vi "ageing subrutine test6.vi"() -> ()   [LabVIEW 2011]
uses:
  <vilib>/Utility/miscctls.llb/LVRowAndColumnTypeDef.ctl
  Controls Win/Control 3.ctl
  <vilib>/Utility/file.llb/Write To Spreadsheet File (string).vi
  <vilib>/Utility/file.llb/Read From Spreadsheet File (string).vi
  <vilib>/regexp/Match Regular Expression.xnode
panel:
  out "Flag 2":bool=TRUE
  out "Flag1":bool=TRUE
  out "Ageing array":string[](array[string])
  out "EditPos Subc":T1
  in  "Ageing Gas":enum32{"Radio Selection 1", "Radio Selection 2"}(radio)
  out "Total Test Duration (Hr)":string
  in  "Clear Pattern":bool
  in  "Clear Pattern":bool
  in  "Subcycle name":string
  in  "Subcycle Pattern":string[][](table) caption="Subcycle pattern"
  in  "stop":bool
  out "Cycle Compiled":bool
  in  "Load cycle for test":bool
  in  "Cycle name":string
  in  "Cycle List":i32(listbox)=2
  in  "Delete Cycle":bool
  in  "Load Cycle":bool
  in  "Save Cycle":bool
  in  "Delete Subcycle":bool
  in  "Subcycle List":i32(listbox)=1
  in  "Load Subcycle":bool
  in  "Save Subcycle":bool
  in  "Cycle Pattern":string[][](table)
  in  "Total Number of Cycles":dbl=1.0 min=1.0
  # "Ageing Program"
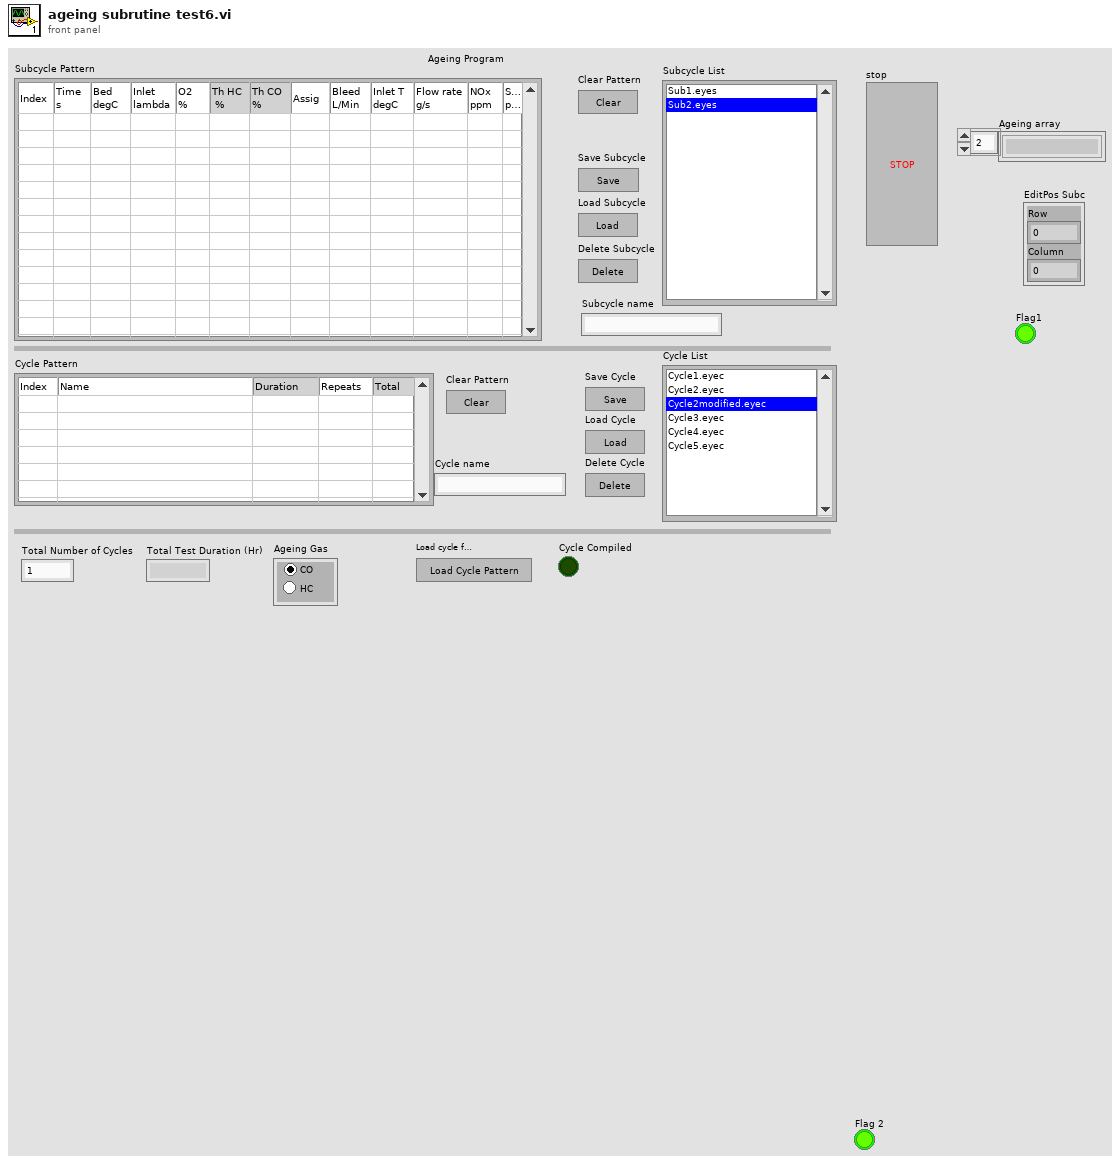
[diagram p1: front panel]
types:
  T1 = typedef "LVRowAndColumnTypeDef.ctl" = cluster{"Row":i32, "Column":i32}
  T2 = typedef "Control 3.ctl" = enum16{"main", "start test", "save subc", "load subc", "delete subc", "clear table 1", "update list 1", "save cycle", "load cycle", "delete cycle", "clear table 2", "update list 2", "calc HC CO", "Total time calc", "update Cycle pattern ", "load cycle name", "convert to num", "load test array", "check scycle name", "check cycle name"}
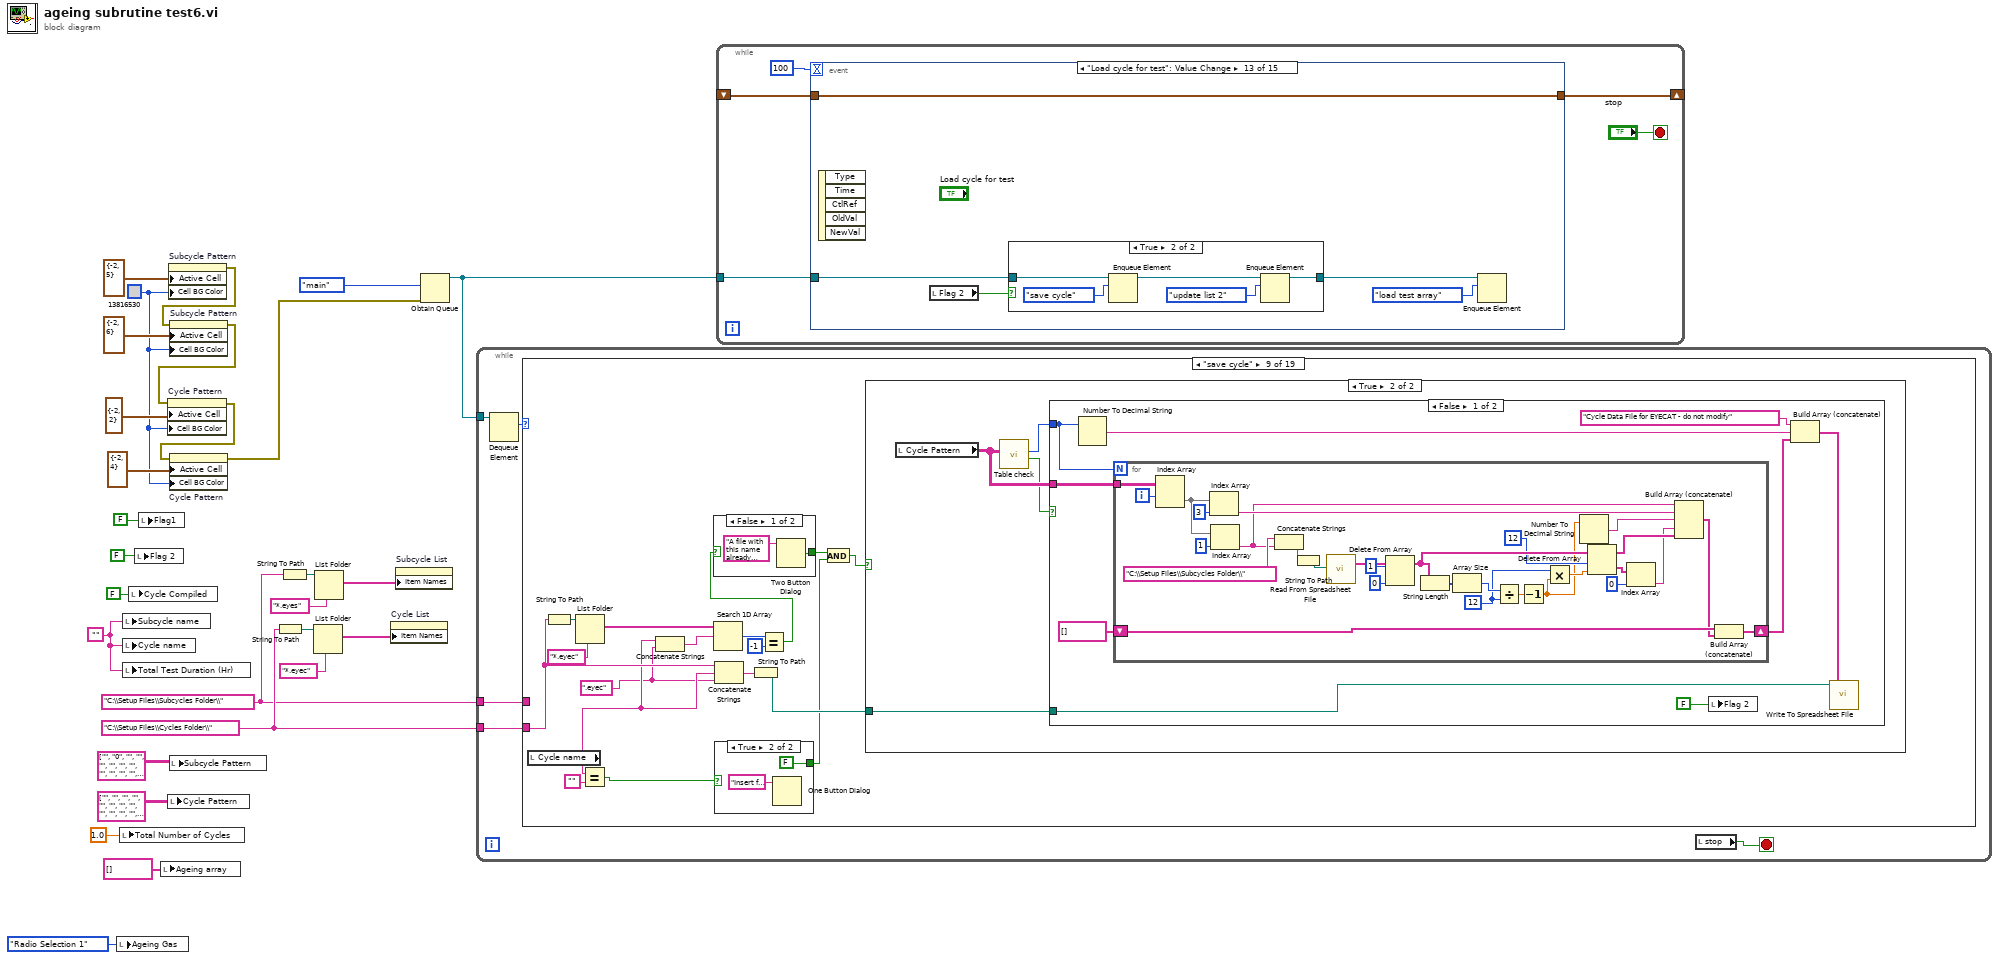
[diagram p0: block diagram]
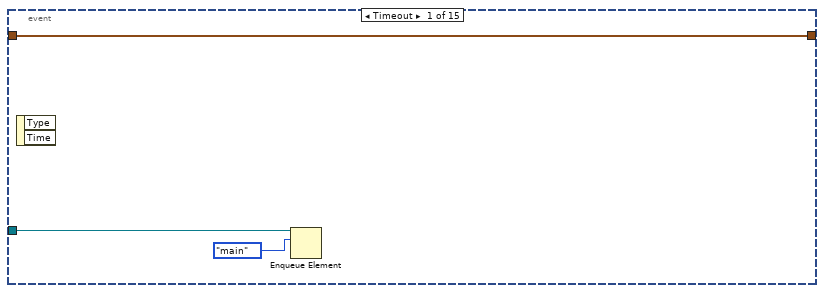
[diagram p2: hidden frame]
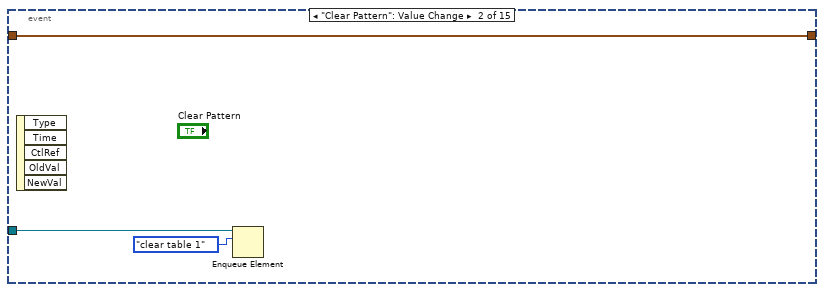
[diagram p3: hidden frame]
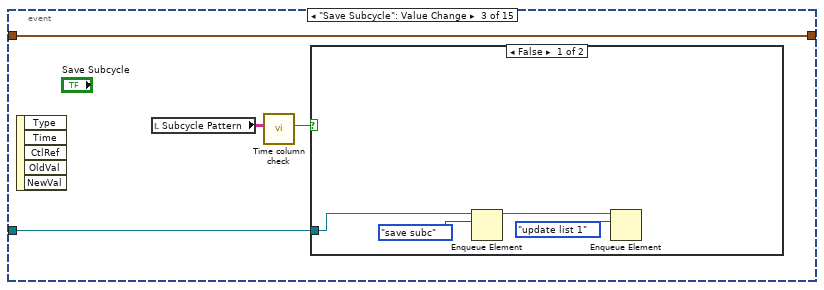
[diagram p4: hidden frame]
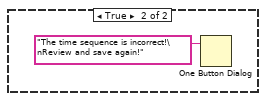
[diagram p5: hidden frame]
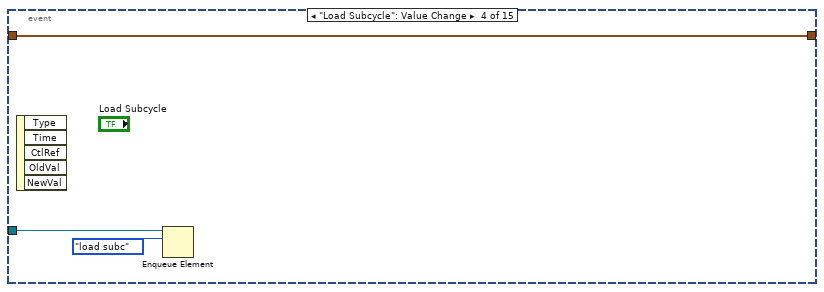
[diagram p6: hidden frame]
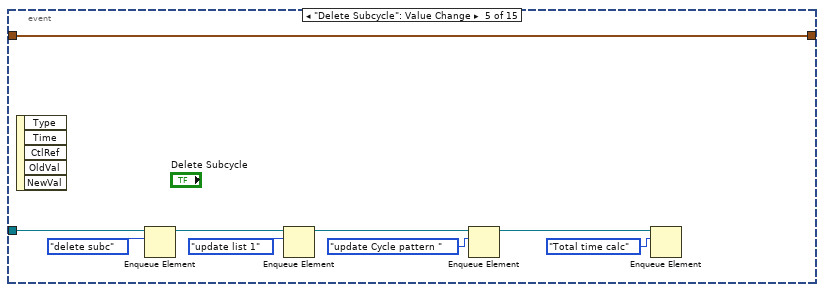
[diagram p7: hidden frame]
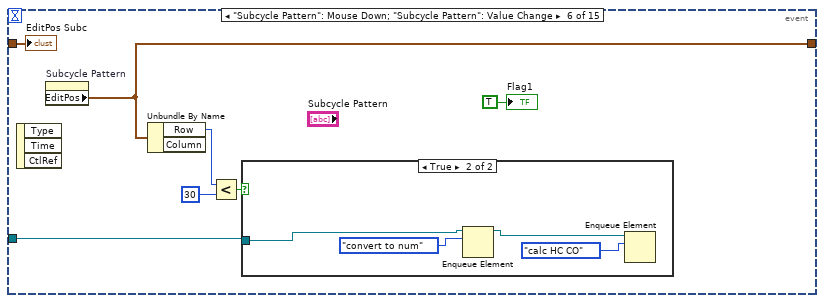
[diagram p8: hidden frame]
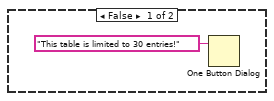
[diagram p9: hidden frame]
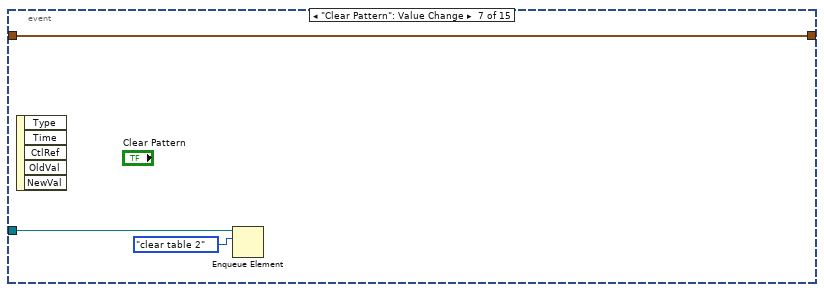
[diagram p10: hidden frame]
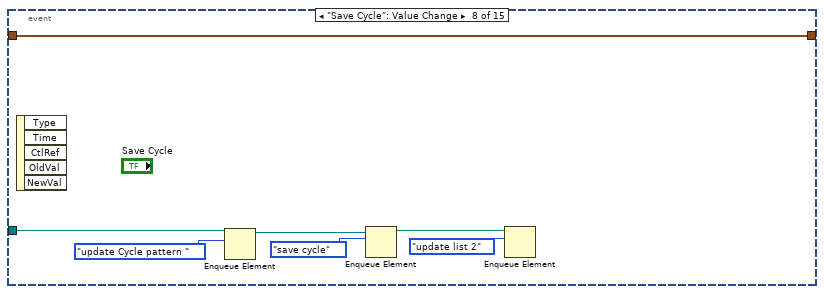
[diagram p11: hidden frame]
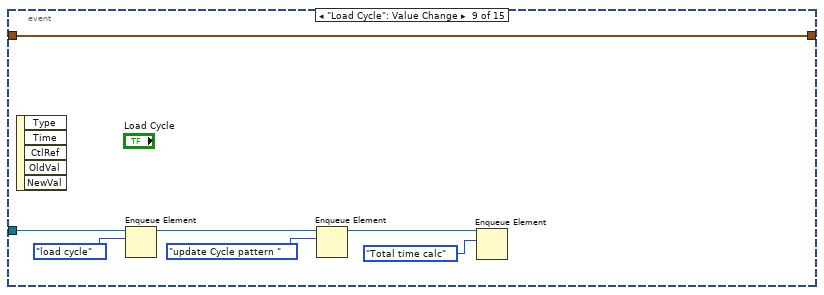
[diagram p12: hidden frame]
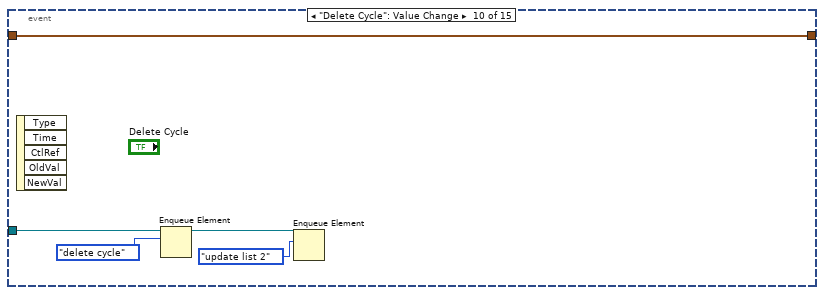
[diagram p13: hidden frame]
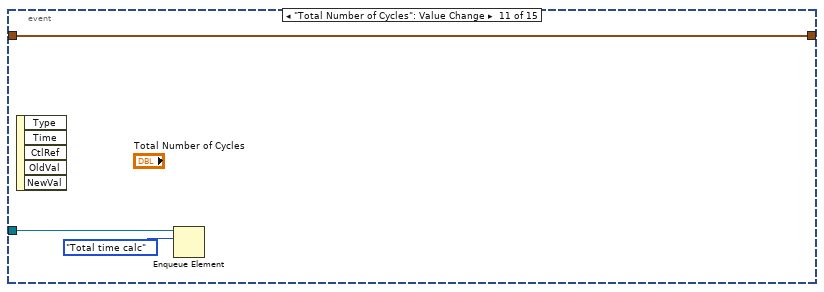
[diagram p14: hidden frame]
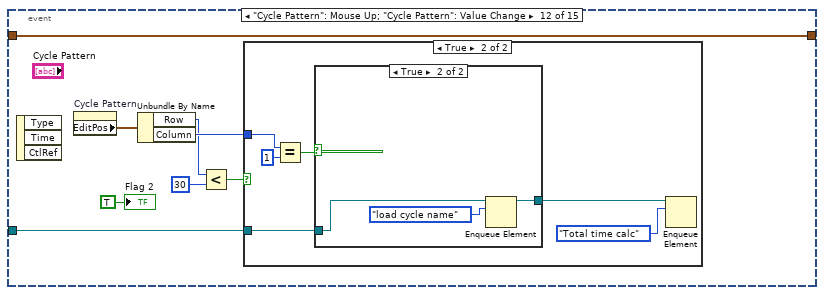
[diagram p15: hidden frame]
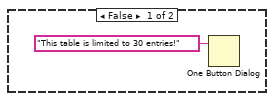
[diagram p16: hidden frame]
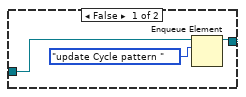
[diagram p17: hidden frame]
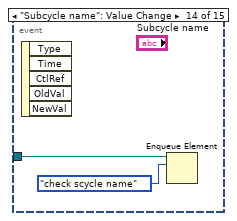
[diagram p19: hidden frame]
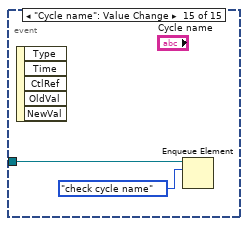
[diagram p20: hidden frame]
diagram:
  w10 = ""
  w13 = "C:\\Setup Files\\Cycles Folder\\"
  w19 = u32 13816530
  w11 = "C:\\Setup Files\\Subcycles Folder\\"
  n1 = local write "Ageing Gas"(enum32{"Radio Selection 1", "Radio Selection 2"}."Radio Selection 1" ("Ageing Gas")) -> ()
  n2 = local write "Total Number of Cycles"(1.0 ("Inlet Temperature (degC)")) -> ()
  n3 = local write "Subcycle name"(w10) -> ()
  n4 = local write "Cycle name"(w10) -> ()
  n5 = local write "Total Test Duration (Hr)"(w10) -> ()
  n6 = local write "Cycle Compiled"(FALSE ("Cycle Compiled")) -> ()
  n7 = local write "Flag 2"(FALSE) -> ()
  n8 = local write "Flag1"(FALSE) -> ()
  n9 = local write "Ageing array"(string[] [] ("Ageing array")) -> ()
  n10 = local write "Cycle Pattern"(string[][] [["", "", "", "", ""], ["", "", "", "", ""], ["", "", "", "", ""], ["", "", "", "", ""], ["", "", "", "", ""], ["", "", "", "", ""], ["", "", "", "", ""], ["", "", "", "", ""], ["", "", "", "", ""], ["", "", "", "", ""], ["", "", "", "", ""], ["", "", "", "", ""], ["", "", "", "", ""], ["", "", "", "", ""], ["", "", "", "", ""], ["", "", "", "", ""], ["", "", "", "", ""], ["", "", "", "", ""], ["", "", "", "", ""], ["", "", "", "", ""], ["", "", "", "", ""], ["", "", "", "", ""], ["", "", "", "", ""], ["", "", "", "", ""], ["", "", "", "", ""], ["", "", "", "", ""], ["", "", "", "", ""], ["", "", "", "", ""], ["", "", "", "", ""], ["", "", "", "", ""], ["", "", "", "", ""]]) -> ()
  n11 = property on="Subcycle Pattern" class="Tbl (strict)"("Active Cell"=T1 {"Row"=-2, "Column"=5} ("Active Cell:Active Cell"), "Cell BG Color"=w19) -> (error out=w24:errorcluster)  [unwired: 2 in, 1 out]
  n12 = property on="Subcycle Pattern" class="Tbl (strict)"(error in=w24, "Active Cell"=T1 {"Row"=-2, "Column"=6} ("Active Cell:Active Cell"), "Cell BG Color"=w19) -> (error out=w23:errorcluster)  [unwired: 1 in, 1 out]
  n13 = property on="Cycle Pattern" class="Tbl (strict)"(error in=w23, "Active Cell"=T1 {"Row"=-2, "Column"=2} ("Active Cell:Active Cell"), "Cell BG Color"=w19) -> (error out=w21:errorcluster)  [unwired: 1 in, 1 out]
  n14 = property on="Cycle Pattern" class="Tbl (strict)"(error in=w21, "Active Cell"=T1 {"Row"=-2, "Column"=4} ("Active Cell:Active Cell"), "Cell BG Color"=w19) -> (error out=w18:errorcluster)  [unwired: 1 in, 1 out]
  n15 = local write "Subcycle Pattern"(string[][] [["", "0", "", "", "", "", "", "", "", "", "", "", ""], ["", "", "", "", "", "", "", "", "", "", "", "", ""], ["", "", "", "", "", "", "", "", "", "", "", "", ""], ["", "", "", "", "", "", "", "", "", "", "", "", ""], ["", "", "", "", "", "", "", "", "", "", "", "", ""], ["", "", "", "", "", "", "", "", "", "", "", "", ""], ["", "", "", "", "", "", "", "", "", "", "", "", ""], ["", "", "", "", "", "", "", "", "", "", "", "", ""], ["", "", "", "", "", "", "", "", "", "", "", "", ""], ["", "", "", "", "", "", "", "", "", "", "", "", ""], ["", "", "", "", "", "", "", "", "", "", "", "", ""], ["", "", "", "", "", "", "", "", "", "", "", "", ""], ["", "", "", "", "", "", "", "", "", "", "", "", ""], ["", "", "", "", "", "", "", "", "", "", "", "", ""], ["", "", "", "", "", "", "", "", "", "", "", "", ""], ["", "", "", "", "", "", "", "", "", "", "", "", ""], ["", "", "", "", "", "", "", "", "", "", "", "", ""], ["", "", "", "", "", "", "", "", "", "", "", "", ""], ["", "", "", "", "", "", "", "", "", "", "", "", ""], ["", "", "", "", "", "", "", "", "", "", "", "", ""], ["", "", "", "", "", "", "", "", "", "", "", "", ""], ["", "", "", "", "", "", "", "", "", "", "", "", ""], ["", "", "", "", "", "", "", "", "", "", "", "", ""], ["", "", "", "", "", "", "", "", "", "", "", "", ""], ["", "", "", "", "", "", "", "", "", "", "", "", ""], ["", "", "", "", "", "", "", "", "", "", "", "", ""], ["", "", "", "", "", "", "", "", "", "", "", "", ""], ["", "", "", "", "", "", "", "", "", "", "", "", ""], ["", "", "", "", "", "", "", "", "", "", "", "", ""], ["", "", "", "", "", "", "", "", "", "", "", "", ""], ["", "", "", "", "", "", "", "", "", "", "", "", ""]]) -> ()
  n16 = String To Path(string=w13) -> (path=w14:path)
  n17 = String To Path(string=w11) -> (path=w16:path)
  n18 = List Folder(path=w14, pattern="*.eyec") -> (filenames=w15:string[])  [unwired: 2 in, 3 out]
  n19 = List Folder(path=w16, pattern="*.eyes") -> (filenames=w17:string[])  [unwired: 2 in, 3 out]
  n20 = property on="Cycle List" class="LstBox (strict)"("Item Names"=w15) -> ()  [unwired: 2 in, 2 out]
  n21 = property on="Subcycle List" class="LstBox (strict)"("Item Names"=w17) -> ()  [unwired: 2 in, 2 out]
  n22 = Obtain Queue(element data type=Control_3."main" ("Enum"), error in (no error)=w18) -> (queue out=w27:refnum<queue>)  [unwired: 3 in, 2 out]
  n23 = while {
    tunnel: w27 -> [w32]
    tunnel: w11 -> [w30]
    tunnel: w13 -> [w29]
    stop <- w33 stop-if-true
    n24 = Dequeue Element(queue=w32) -> (element=w31:T2)  [unwired: 2 in, 3 out]
    n25 = case shown="\"save cycle\"" w31 {
      tunnel: w30 -> [_ _ w40 w51 w87 w121 _ _ _ _ _ _ _ w464 _ _ _ _ _]
      tunnel: w29 -> [_ _ _ _ _ _ _ w134 w149 w204 w249 _ _ _ _ _ _ _ _]
      frame "main", Default {
      }
      frame "clear table 1" {
        n26 = property on="Subcycle name" class="Str"("Value"="" ("Subcycle name")) -> ()  [unwired: 2 in, 2 out]
        n27 = local write "Flag1"(FALSE) -> ()
        n28 = local write "Subcycle Pattern"(string[][] [["", "0", "", "", "", "", "", "", "", "", "", "", ""], ["", "", "", "", "", "", "", "", "", "", "", "", ""], ["", "", "", "", "", "", "", "", "", "", "", "", ""], ["", "", "", "", "", "", "", "", "", "", "", "", ""], ["", "", "", "", "", "", "", "", "", "", "", "", ""], ["", "", "", "", "", "", "", "", "", "", "", "", ""], ["", "", "", "", "", "", "", "", "", "", "", "", ""], ["", "", "", "", "", "", "", "", "", "", "", "", ""], ["", "", "", "", "", "", "", "", "", "", "", "", ""], ["", "", "", "", "", "", "", "", "", "", "", "", ""], ["", "", "", "", "", "", "", "", "", "", "", "", ""], ["", "", "", "", "", "", "", "", "", "", "", "", ""], ["", "", "", "", "", "", "", "", "", "", "", "", ""], ["", "", "", "", "", "", "", "", "", "", "", "", ""], ["", "", "", "", "", "", "", "", "", "", "", "", ""], ["", "", "", "", "", "", "", "", "", "", "", "", ""], ["", "", "", "", "", "", "", "", "", "", "", "", ""], ["", "", "", "", "", "", "", "", "", "", "", "", ""], ["", "", "", "", "", "", "", "", "", "", "", "", ""], ["", "", "", "", "", "", "", "", "", "", "", "", ""], ["", "", "", "", "", "", "", "", "", "", "", "", ""], ["", "", "", "", "", "", "", "", "", "", "", "", ""], ["", "", "", "", "", "", "", "", "", "", "", "", ""], ["", "", "", "", "", "", "", "", "", "", "", "", ""], ["", "", "", "", "", "", "", "", "", "", "", "", ""], ["", "", "", "", "", "", "", "", "", "", "", "", ""], ["", "", "", "", "", "", "", "", "", "", "", "", ""], ["", "", "", "", "", "", "", "", "", "", "", "", ""], ["", "", "", "", "", "", "", "", "", "", "", "", ""], ["", "", "", "", "", "", "", "", "", "", "", "", ""], ["", "", "", "", "", "", "", "", "", "", "", "", ""]]) -> ()
      }
      frame "update list 1" {
        n29 = String To Path(string=w40) -> (path=w39:path)
        n30 = List Folder(path=w39, pattern="*.eyes") -> (filenames=w38:string[])  [unwired: 2 in, 3 out]
        n31 = property on="Subcycle List" class="LstBox (strict)"("Item Names"=w38) -> ()  [unwired: 2 in, 2 out]
      }
      frame "save subc" {
        w44 = ".eyes" ("string")
        n32 = local read "Subcycle name"() -> (w43:string)
        n33 = String To Path(string=w51) -> (path=w56:path)
        n34 = Equal?(x=w43, y="") -> (x = y?=w48:bool)
        n35 = List Folder(path=w56, pattern="*.eyes" ("string")) -> (filenames=w55:string[])  [unwired: 2 in, 3 out]
        n36 = Concatenate Strings(w43, w44) -> (w42:string)
        n37 = Concatenate Strings(w51, w43, w44) -> (w57:string)
        n38 = Search 1D Array(1D array=w55, element=w42) -> (index of element=w54:i32)  [unwired: 1 in]
        n39 = case shown="True" w48 {
          tunnel: [TRUE FALSE] -> w47
          frame False {
          }
          frame True {
            n40 = One Button Dialog(message="Insert file name!") -> ()  [unwired: 1 in, 1 out]
          }
        }
        n41 = String To Path(string=w57) -> (path=w50:path)
        n42 = Equal?(x=w54, y=-1) -> (x = y?=w52:bool)
        n43 = case shown="False" w52 {
          selector: w52 -> [_ w63]
          tunnel: [w61 w63] -> w46
          frame False {
            n44 = Two Button Dialog(message="A file with this name already exists!\nDo you want to overwrite?") -> (T button?=w61:bool)  [unwired: 2 in]
          }
          frame True {
          }
        }
        n45 = And(x=w46, y=w47) -> (x .and. y?=w45:bool)
        n46 = case shown="True" w45 {
          tunnel: w50 -> [_ w68]
          frame False {
          }
          frame True {
            n47 = local read "Subcycle Pattern"() -> (w67:string[][])
            n48 = call "Table check.vi"("Input table"=w67) -> ("Incomplete?"=w65:bool, "Length"=w66:i32)  [unwired: 9 in]
            n49 = case shown="False" w65 {
              tunnel: w67 -> [w76 _]
              tunnel: w68 -> [w75 _]
              tunnel: w66 -> [w74 _]
              tunnel: string[] [] -> [w73 _]
              frame False {
                n50 = for {
                  N: w74 -> [_]
                  tunnel: w76 -> [w83]
                  shift-right: [w80] -> w72
                  shift-left: w73 -> [w81]
                  i -> [w82]
                  n51 = Index Array(array=w83, index (row)=w82) -> (element=w79:string[])  [unwired: 1 in]
                  n52 = Delete From Array(array=w79, index=0) -> (array with subset deleted=w78:string[])  [unwired: 1 in, 1 out]
                  n53 = Build Array (concatenate)(w81, w78) -> (w80:string[])
                }
                n54 = Build Array (concatenate)("SubCycle Data File for EYECAT - do not modify", w72) -> (w70:string[])
                n55 = call-poly <vilib>:"Write To Spreadsheet File.vi"("1D data"=w70, "file path (dialog if empty)"=w75) -> ()  [unwired: 6 in, 1 out]
              }
              frame True {
                n56 = One Button Dialog(message="The table is incomplete!\nplease review and save again!") -> ()  [unwired: 1 in, 1 out]
              }
            }
            n57 = local write "Flag1"(FALSE) -> ()
          }
        }
      }
      frame "load subc" {
        n58 = local read "Flag1"() -> (w88:bool)
        n59 = case shown="True" w88 {
          tunnel: [w115 w117] -> w86
          tunnel: w87 -> [w115 w117]
          tunnel: [TRUE w116] -> w85
          frame False {
          }
          frame True {
            n60 = Two Button Dialog(message="The table has been modified.\nDo you want to continue?") -> (T button?=w116:bool)  [unwired: 2 in]
          }
        }
        n61 = case shown="True" w85 {
          tunnel: w86 -> [_ w92]
          frame False {
          }
          frame True {
            n62 = property on="Subcycle List" class="LstBox (strict)"() -> ("Item Names"=w104:string[])  [unwired: 2 in, 2 out]
            n63 = Index Array(array=w104, index="Subcycle List") -> (element=w91:string)
            n64 = Concatenate Strings(w92, w91) -> (w102:string)
            n65 = Search/Split String(string=w91, search string/char (-)=".") -> (substring before match=w89:string)  [unwired: 1 in, 2 out]
            n66 = String To Path(string=w102) -> (path=w101:path)
            n67 = local write "Subcycle name"(w89) -> ()
            n68 = call-poly <vilib>:"Read From Spreadsheet File.vi"("file path (dialog if empty)"=w101) -> ("first row"=w97:string[])  [unwired: 6 in, 4 out]
            n69 = Delete From Array(array=w97, length=1, index=0) -> (array with subset deleted=w94:string[])  [unwired: 1 out]
            n70 = Array Size(array=w94) -> (size(s)=w100:i32)
            n71 = Divide(x=w100, y=12) -> (x/y=w93:dbl)
            n72 = for {
              N: w93 -> [_]
              shift-right: [w110] -> _
              shift-left: w94 -> [w113]
              tunnel: [w109] -> w98 mode=indexing
              i -> [w108]
              n73 = Increment(x=w108) -> (x+1=w107:i32)
              n74 = Delete From Array(array=w113, length=12, index=0) -> (deleted portion=w105:string[], array with subset deleted=w110:string[])
              n75 = Number To Decimal String(number=w107) -> (decimal integer string=w106:string)  [unwired: 1 in]
              n76 = Build Array (concatenate)(w106, w105) -> (w109:string[])
            }
            n77 = local write "Subcycle Pattern"(w98) -> ()
          }
        }
      }
      frame "delete subc" {
        n78 = Two Button Dialog(message="This operation will permanently delete this file!\nDo you want to continue?") -> (T button?=w120:bool)  [unwired: 2 in]
        n79 = case shown="True" w120 {
          tunnel: w121 -> [_ w126]
          frame False {
          }
          frame True {
            n80 = local read "Subcycle List"() -> (w123:i32)
            n81 = property on="Subcycle List" class="LstBox (strict)"() -> ("Item Names"=w124:string[])  [unwired: 2 in, 2 out]
            n82 = Index Array(array=w124, index=w123) -> (element=w128:string)
            n83 = Concatenate Strings(w126, w128) -> (w127:string)
            n84 = local write "Flag1"(FALSE) -> ()
            n85 = String To Path(string=w127) -> (path=w125:path)
            n86 = Delete(path (use dialog)=w125) -> ()  [unwired: 4 in, 3 out]
          }
        }
      }
      frame "clear table 2" {
        n87 = property on="Cycle name" class="Str"("Value"="" ("Subcycle name")) -> ()  [unwired: 2 in, 2 out]
        n88 = local write "Flag 2"(FALSE) -> ()
        n89 = local write "Cycle Pattern"(string[][] [["", "", "", "", ""], ["", "", "", "", ""], ["", "", "", "", ""], ["", "", "", "", ""], ["", "", "", "", ""], ["", "", "", "", ""], ["", "", "", "", ""], ["", "", "", "", ""], ["", "", "", "", ""], ["", "", "", "", ""], ["", "", "", "", ""], ["", "", "", "", ""], ["", "", "", "", ""], ["", "", "", "", ""], ["", "", "", "", ""], ["", "", "", "", ""], ["", "", "", "", ""], ["", "", "", "", ""], ["", "", "", "", ""], ["", "", "", "", ""], ["", "", "", "", ""], ["", "", "", "", ""], ["", "", "", "", ""], ["", "", "", "", ""], ["", "", "", "", ""], ["", "", "", "", ""], ["", "", "", "", ""], ["", "", "", "", ""], ["", "", "", "", ""], ["", "", "", "", ""], ["", "", "", "", ""]]) -> ()
      }
      frame "update list 2" {
        n90 = String To Path(string=w134) -> (path=w135:path)
        n91 = List Folder(path=w135, pattern="*.eyec") -> (filenames=w133:string[])  [unwired: 2 in, 3 out]
        n92 = property on="Cycle List" class="LstBox (strict)"("Item Names"=w133) -> ()  [unwired: 2 in, 2 out]
      }
      frame "save cycle" {
        w136 = ".eyec" ("string")
        n93 = local read "Cycle name"() -> (w137:string)
        n94 = String To Path(string=w149) -> (path=w150:path)
        n95 = List Folder(path=w150, pattern="*.eyec" ("string")) -> (filenames=w148:string[])  [unwired: 2 in, 3 out]
        n96 = Equal?(x=w137, y="") -> (x = y?=w143:bool)
        n97 = Concatenate Strings(w137, w136) -> (w139:string)
        n98 = Search 1D Array(1D array=w148, element=w139) -> (index of element=w147:i32)  [unwired: 1 in]
        n99 = Concatenate Strings(w149, w137, w136) -> (w152:string)
        n100 = case shown="True" w143 {
          tunnel: [TRUE FALSE] -> w141
          frame False {
          }
          frame True {
            n101 = One Button Dialog(message="Insert file name!") -> ()  [unwired: 1 in, 1 out]
          }
        }
        n102 = String To Path(string=w152) -> (path=w151:path)
        n103 = Equal?(x=w147, y=-1) -> (x = y?=w145:bool)
        n104 = case shown="False" w145 {
          selector: w145 -> [_ w201]
          tunnel: [w199 w201] -> w142
          frame False {
            n105 = Two Button Dialog(message="A file with this name already exists!\nDo you want to overwrite?") -> (T button?=w199:bool)  [unwired: 2 in]
          }
          frame True {
          }
        }
        n106 = And(x=w142, y=w141) -> (x .and. y?=w140:bool)
        n107 = case shown="True" w140 {
          tunnel: w151 -> [_ w159]
          frame False {
          }
          frame True {
            n108 = local read "Cycle Pattern"() -> (w158:string[][])
            n109 = call "Table check.vi"("Input table"=w158) -> ("Incomplete?"=w156:bool, "Length"=w157:i32)  [unwired: 9 in]
            n110 = case shown="False" w156 {
              tunnel: w159 -> [w168 _]
              tunnel: w158 -> [w167 _]
              tunnel: w157 -> [w160 _]
              frame False {
                n111 = Number To Decimal String(number=w160) -> (decimal integer string=w163:string)  [unwired: 1 in]
                n112 = for {
                  N: w160 -> [_]
                  tunnel: w167 -> [w197]
                  shift-right: [w185] -> w164
                  shift-left: string[] [] -> [w195]
                  i -> [w196]
                  w176 = 12 ("length")
                  n113 = Index Array(array=w197, index (row)=w196) -> (element=w191:string[])  [unwired: 1 in]
                  n114 = Index Array(array=w191, index=3) -> (element=w181:string)
                  n115 = Index Array(array=w191, index=1) -> (element=w180:string)
                  n116 = Concatenate Strings("C:\\Setup Files\\Subcycles Folder\\", w180) -> (w192:string)
                  n117 = String To Path(string=w192) -> (path=w193:path)
                  n118 = call-poly <vilib>:"Read From Spreadsheet File.vi"("file path (dialog if empty)"=w193) -> ("first row"=w184:string[])  [unwired: 6 in, 4 out]
                  n119 = Delete From Array(array=w184, length=1, index=0) -> (array with subset deleted=w178:string[])  [unwired: 1 out]
                  n120 = String Length(string=w178) -> (length=w187:i32[])
                  n121 = Array Size(array=w187) -> (size(s)=w179:i32)
                  n122 = Divide(x=w179, y=w176) -> (x/y=w177:dbl)
                  n123 = Decrement(x=w177) -> (x-1=w169:dbl)
                  n124 = Multiply(x=w176, y=w169) -> (x*y=w175:dbl)
                  n125 = Number To Decimal String(number=w169) -> (decimal integer string=w186:string)  [unwired: 1 in]
                  n126 = Delete From Array(array=w178, length=12, index=w175) -> (deleted portion=w172:string[], array with subset deleted=w173:string[])
                  n127 = Index Array(array=w172, index=0) -> (element=w170:string)
                  n128 = Build Array (concatenate)(w180, w181, w186, w170, w173) -> (w190:string[])
                  n129 = Build Array (concatenate)(w195, w190) -> (w185:string[])
                }
                n130 = local write "Flag 2"(FALSE) -> ()
                n131 = Build Array (concatenate)("Cycle Data File for EYECAT - do not modify", w163, w164) -> (w165:string[])
                n132 = call-poly <vilib>:"Write To Spreadsheet File.vi"("1D data"=w165, "file path (dialog if empty)"=w168) -> ()  [unwired: 6 in, 1 out]
              }
              frame True {
                n133 = One Button Dialog(message="The table is incomplete!\nplease review and save again!") -> ()  [unwired: 1 in, 1 out]
              }
            }
          }
        }
      }
      frame "load cycle" {
        n134 = local read "Flag 2"() -> (w205:bool)
        n135 = case shown="False" w205 {
          tunnel: [w244 w246] -> w202
          tunnel: w204 -> [w244 w246]
          tunnel: [TRUE ("T button?") w245] -> w203
          frame False {
          }
          frame True {
            n136 = Two Button Dialog(message="The table has been modified.\nDo you want to continue?") -> (T button?=w245:bool)  [unwired: 2 in]
          }
        }
        n137 = case shown="True" w203 {
          tunnel: w202 -> [_ w208]
          frame False {
          }
          frame True {
            n138 = property on="Cycle List" class="LstBox (strict)"() -> ("Item Names"=w224:string[])  [unwired: 2 in, 2 out]
            n139 = Index Array(array=w224, index="Cycle List") -> (element=w210:string)
            n140 = Concatenate Strings(w208, w210) -> (w223:string)
            n141 = Search/Split String(string=w210, search string/char (-)=".") -> (substring before match=w209:string)  [unwired: 1 in, 2 out]
            n142 = String To Path(string=w223) -> (path=w222:path)
            n143 = local write "Cycle name"(w209) -> ()
            n144 = call-poly <vilib>:"Read From Spreadsheet File.vi"("file path (dialog if empty)"=w222) -> ("first row"=w206:string[])  [unwired: 6 in, 4 out]
            n145 = Delete From Array(array=w206, length=2, index=0) -> (array with subset deleted=w207:string[])  [unwired: 1 out]
            n146 = Index Array(array=w206, index=1) -> (element=w221:string)
            n147 = Decimal String To Number(string=w221) -> (number=w220:i32)  [unwired: 2 in, 1 out]
            n148 = for {
              N: w220 -> [_]
              tunnel: w207 -> [w242]
              tunnel: [w237] -> w215 mode=indexing
              shift-right: [w227] -> _
              shift-left: 0 ("x") -> [w228]
              i -> [w241]
              w238 = ""
              n149 = Increment(x=w228) -> (x+1=w226:i32)
              n150 = Increment(x=w226) -> (x+1=w234:i32)
              n151 = Increment(x=w241) -> (x+1=w236:i32)
              n152 = Number To Decimal String(number=w236) -> (decimal integer string=w235:string)  [unwired: 1 in]
              n153 = Index Array(array=w242, index #1=w228, index #2=w226, index #3=w234) -> (element #1=w240:string, element #2=w239:string, element #3=w233:string)
              n154 = Build Array(w235, w240, w238, w239, w238) -> (w237:string[])
              n155 = Decimal String To Number(string=w233) -> (number=w232:i32)  [unwired: 2 in, 1 out]
              n156 = Multiply(x=w232, y=12 ("x")) -> (x*y=w230:i32)
              n157 = Compound Arithmetic op=ADD(w230, 4, w228) -> (w227:i32)
            }
            n158 = Insert Into Array(array=string[][] [["", "", "", "", ""], ["", "", "", "", ""], ["", "", "", "", ""], ["", "", "", "", ""], ["", "", "", "", ""], ["", "", "", "", ""], ["", "", "", "", ""], ["", "", "", "", ""], ["", "", "", "", ""], ["", "", "", "", ""], ["", "", "", "", ""], ["", "", "", "", ""], ["", "", "", "", ""], ["", "", "", "", ""], ["", "", "", "", ""], ["", "", "", "", ""], ["", "", "", "", ""], ["", "", "", "", ""], ["", "", "", "", ""], ["", "", "", "", ""], ["", "", "", "", ""], ["", "", "", "", ""], ["", "", "", "", ""], ["", "", "", "", ""], ["", "", "", "", ""], ["", "", "", "", ""], ["", "", "", "", ""], ["", "", "", "", ""], ["", "", "", "", ""], ["", "", "", "", ""], ["", "", "", "", ""]], index (row)=0, new element=w215) -> (w214:string[][])  [unwired: 1 in]
            n159 = local write "Cycle Pattern"(w214) -> ()
          }
        }
      }
      frame "delete cycle" {
        n160 = Two Button Dialog(message="This operation will permanently delete this file!\nDo you want to continue?") -> (T button?=w250:bool)  [unwired: 2 in]
        n161 = case shown="True" w250 {
          tunnel: w249 -> [_ w255]
          frame False {
          }
          frame True {
            n162 = local read "Cycle List"() -> (w256:i32)
            n163 = property on="Cycle List" class="LstBox (strict)"() -> ("Item Names"=w257:string[])  [unwired: 2 in, 2 out]
            n164 = Index Array(array=w257, index=w256) -> (element=w254:string)
            n165 = Concatenate Strings(w255, w254) -> (w253:string)
            n166 = String To Path(string=w253) -> (path=w252:path)
            n167 = Delete(path (use dialog)=w252) -> ()  [unwired: 4 in, 3 out]
            n168 = local write "Flag 2"(FALSE) -> ()
          }
        }
      }
      frame "calc HC CO" {
        n169 = local read "Subcycle Pattern"() -> (w272:string[][])
        n170 = Index Array(array=w272, index (col) #1=3 ("disabled index (col)"), index (col) #2=4 ("index (col)")) -> (element #1=w262:string[], element #2=w269:string[])  [unwired: 2 in]
        n171 = Array Size(array=w262) -> (size(s)=w260:i32)
        n172 = Search 1D Array(1D array=w262, element="") -> (index of element=w259:i32)  [unwired: 1 in]
        n173 = Equal?(x=w259, y=-1) -> (x = y?=w261:bool)
        n174 = Select(t=w260, s=w261, f=w259) -> (s? t:f=w258:i32)
        n175 = for {
          N: w258 -> [_]
          tunnel: [w277] -> w266 mode=indexing
          tunnel: [w276] -> w265 mode=indexing
          tunnel: w262 -> [w275] mode=indexing
          tunnel: w269 -> [w274] mode=indexing
          w281 = ""
          # "update the equations!!!!"
          n176 = Not Equal?(x=w275, y=w281) -> (x != y?=w280:bool)
          n177 = Not Equal?(x=w274, y=w281) -> (x != y?=w279:bool)
          n178 = And(x=w280, y=w279) -> (x .and. y?=w278:bool)
          n179 = case shown="True" w278 {
            tunnel: w275 -> [_ w294]
            tunnel: w274 -> [_ w293]
            tunnel: [w282 w287] -> w276
            tunnel: [w282 w285] -> w277
            frame False {
              w282 = ""
            }
            frame True {
              n180 = Fract/Exp String To Number(string=w294) -> (number=w292:dbl)  [unwired: 3 in, 1 out]
              n181 = Fract/Exp String To Number(string=w293) -> (number=w291:dbl)  [unwired: 3 in, 1 out]
              n182 = Add(x=w292, y=w291) -> (x+y=w286:dbl)
              n183 = Subtract(x=w292, y=w291) -> (x-y=w288:dbl)
              n184 = Number To Fractional String(number=w286, width (-)=i16 3, precision (6)=i16 1) -> (F-format string=w285:string)  [unwired: 1 in]
              n185 = Number To Fractional String(number=w288, width (-)=i16 3, precision (6)=i16 1) -> (F-format string=w287:string)  [unwired: 1 in]
            }
          }
        }
        n186 = Replace Array Subset(array=w272, new element #1=w266, index (col) #1=5 ("disabled index (col)"), new element #2=w265, index (col) #2=6 ("disabled index (col)")) -> (w270:string[][])  [unwired: 2 in]
        n187 = local write "Subcycle Pattern"(w270) -> ()
      }
      frame "Total time calc" {
        w309 = i16 2 ("width (-)")
        w316 = ":"
        n188 = local read "Cycle Pattern"() -> (w323:string[][])
        n189 = Index Array(array=w323, index (col)=4 ("disabled index (col)")) -> (element=w296:string[])  [unwired: 1 in]
        n190 = Array Size(array=w296) -> (size(s)=w298:i32)
        n191 = Search 1D Array(1D array=w296, element="") -> (index of element=w297:i32)  [unwired: 1 in]
        n192 = Equal?(x=w297, y=-1) -> (x = y?=w299:bool)
        n193 = Select(t=w298, s=w299, f=w297) -> (s? t:f=w295:i32)
        n194 = for {
          N: w295 -> [_]
          tunnel: w296 -> [w331] mode=indexing
          shift-right: [w333] -> w319
          shift-left: 0 -> [w334]
          n195 = xnode "Match Regular Expression"("input string"=w331, "regular expression"=":" ("search string/char (-)")) -> ("before match"=w330:string, "after match"=w327:string)  [unwired: 4 in, 3 out]
          n196 = Decimal String To Number(string=w330) -> (number=w329:i32)  [unwired: 2 in, 1 out]
          n197 = Decimal String To Number(string=w327) -> (number=w326:i32)  [unwired: 2 in, 1 out]
          n198 = Multiply(x=w329, y=60) -> (x*y=w325:i32)
          n199 = Add(x=w325, y=w326) -> (x+y=w324:i32)
          n200 = Add(x=w324, y=w334) -> (x+y=w333:i32)
        }
        n201 = local read "Total Number of Cycles"() -> (w320:dbl)
        n202 = Multiply(x=w319, y=w320) -> (x*y=w315:dbl)
        n203 = Quotient & Remainder(x=w315, y=3600.0) -> (x-y*floor(x/y)=w302:dbl, floor(x/y)=w312:dbl)
        n204 = Quotient & Remainder(x=w302, y=60.0) -> (x-y*floor(x/y)=w310:dbl, floor(x/y)=w311:dbl)
        n205 = Number To Decimal String(number=w312) -> (decimal integer string=w317:string)  [unwired: 1 in]
        n206 = Number To Decimal String(number=w311, width (-)=w309) -> (decimal integer string=w313:string)
        n207 = Number To Decimal String(number=w310, width (-)=w309) -> (decimal integer string=w308:string)
        n208 = Concatenate Strings(w317, w316, w313, w316, w308) -> (w307:string)
        n209 = call <vilib>:"Search and Replace Pattern.vi"("string"=w307, "regular expression (\"\")"=" " ("replace string (\"\")"), "replace string (\"\")"="0" ("replace string (\"\")"), "replace all? (F)"=TRUE) -> ("result string"=→"Total Test Duration (Hr)":string)  [unwired: 1 in, 1 out]
      }
      frame "update Cycle pattern " {
        n210 = local read "Cycle Pattern"() -> (w462:string[][])
        n211 = Index Array(array=w462, index (col)=1 ("disabled index (col)")) -> (element=w447:string[])  [unwired: 1 in]
        n212 = String To Path(string=w464) -> (path=w465:path)
        n213 = Array Size(array=w447) -> (size(s)=w450:i32)
        n214 = Search 1D Array(1D array=w447, element="") -> (index of element=w449:i32)  [unwired: 1 in]
        n215 = List Folder(path=w465, pattern="*.eyes") -> (filenames=w463:string[])  [unwired: 2 in, 3 out]
        n216 = Equal?(x=w449, y=-1) -> (x = y?=w451:bool)
        n217 = Select(t=w450, s=w451, f=w449) -> (s? t:f=w448:i32)
        n218 = for {
          N: w448 -> [_]
          tunnel: w462 -> [w481] mode=indexing
          tunnel: w464 -> [w474]
          tunnel: [w476] -> w457 mode=indexing
          tunnel: [w478] -> w461 mode=indexing
          tunnel: [w475] -> w458 mode=indexing
          tunnel: w463 -> [w473]
          tunnel: [w468] -> w454 mode=indexing
          n219 = Index Array(array=w481, index #1=1 ("index"), index #2=3 ("index")) -> (element #1=w472:string, element #2=w477:string)
          n220 = Search 1D Array(1D array=w473, element=w472) -> (index of element=w471:i32)  [unwired: 1 in]
          n221 = Not Equal?(x=w471, y=-1) -> (x != y?=w469:bool)
          n222 = case shown="True" w469 {
            tunnel: [w485 w499] -> w478
            tunnel: w477 -> [_ w495]
            tunnel: [w485 w493] -> w476
            tunnel: [w485 w492] -> w475
            tunnel: w474 -> [_ w491]
            tunnel: w472 -> [w484 w490]
            tunnel: [w483 w490] -> w468
            frame False {
              w485 = "N/A" ("String")
              n223 = Concatenate Strings(w484, " - File NOT AVAILABLE !!!" ("string")) -> (w483:string)
            }
            frame True {
              w503 = i16 2 ("width (-)")
              n224 = Concatenate Strings(w491, w490) -> (w521:string)
              n225 = String To Path(string=w521) -> (path=w520:path)
              n226 = call <vilib>:"Search and Replace Pattern.vi"("string"=w495, "regular expression (\"\")"="[a-x ]" ("format string"), "replace string (\"\")"="", "replace all? (F)"=TRUE) -> ("result string"=w492:string)  [unwired: 1 in, 1 out]
              n227 = call-poly <vilib>:"Read From Spreadsheet File.vi"("file path (dialog if empty)"=w520) -> ("first row"=w489:string[])  [unwired: 6 in, 4 out]
              n228 = Delete From Array(array=w489, length=1, index=0) -> (array with subset deleted=w488:string[])  [unwired: 1 out]
              n229 = Array Size(array=w488) -> (size(s)=w519:i32)
              n230 = Equal?(x=w492, y="") -> (x = y?=w507:bool)
              n231 = Subtract(x=w519, y=12) -> (x-y=w517:i32)
              n232 = Select(t="0", s=w507, f=w492) -> (s? t:f=w506:string)
              n233 = Index Array(array=w488, index=w517) -> (element=w493:string)
              n234 = Decimal String To Number(string=w506) -> (number=w516:i32)  [unwired: 2 in, 1 out]
              n235 = Decimal String To Number(string=w493) -> (number=w515:i32)  [unwired: 2 in, 1 out]
              n236 = Multiply(x=w516, y=w515) -> (x*y=w514:i32)
              n237 = Quotient & Remainder(x=w514, y=60) -> (x-y*floor(x/y)=w512:i32, floor(x/y)=w511:i32)
              n238 = Number To Decimal String(number=w512, width (-)=w503) -> (decimal integer string=w509:string)
              n239 = Number To Decimal String(number=w511, width (-)=w503) -> (decimal integer string=w508:string)
              n240 = Concatenate Strings(w508, ":", w509) -> (w502:string)
              n241 = call <vilib>:"Search and Replace Pattern.vi"("string"=w502, "regular expression (\"\")"=" " ("replace string (\"\")"), "replace string (\"\")"="0" ("replace string (\"\")"), "replace all? (F)"=TRUE) -> ("result string"=w499:string)  [unwired: 1 in, 1 out]
            }
          }
        }
        n242 = Replace Array Subset(array=w462, new element #1=w454, index (col) #1=1 ("disabled index (col)"), new element #2=w457, index (col) #2=2 ("disabled index (col)"), new element #3=w458, index (col) #3=3 ("disabled index (col)"), new element #4=w461, index (col) #4=4 ("disabled index (col)")) -> (w466:string[][])  [unwired: 4 in]
        n243 = local write "Cycle Pattern"(w466) -> ()
      }
      frame "load cycle name" {
        n244 = property on="Cycle Pattern" class="Tbl (strict)"() -> ("EditPos"=w527:T1)  [unwired: 2 in, 2 out]
        n245 = Unbundle By Name(w527) -> ("Row"=w525:i32, "Column"=w524:i32)
        n246 = local read "Cycle Pattern"() -> (w523:string[][])
        n247 = call "SubCycles list.vi"() -> ("Subcycle name"=w526:string)  [unwired: 10 in, 1 out]
        n248 = Replace Array Subset(array=w523, new element=w526, index (row)=w525, index (col)=w524) -> (w522:string[][])
        n249 = local write "Cycle Pattern"(w522) -> ()
      }
      frame "load test array" {
        n250 = local read "Total Test Duration (Hr)"() -> (w530:string)
        n251 = Not Equal?(x=w530, y="0:00:00") -> (x != y?=w528:bool)
        n252 = case shown="True" w528 {
          selector: w528 -> [w532 _]
          tunnel: [FALSE TRUE] -> w531
          frame False {
            n253 = case shown="True" w532 {
              frame False {
                n254 = One Button Dialog(message="The test is empty!\nReview the cycle pattern!") -> ()  [unwired: 1 in, 1 out]
              }
              frame True {
              }
            }
          }
          frame True {
            n255 = local read "Cycle name"() -> (w546:string)
            n256 = Concatenate Strings("C:\\Setup Files\\Cycles Folder\\", w546, ".eyec" ("string")) -> (w544:string)
            n257 = String To Path(string=w544) -> (path=w545:path)
            n258 = local read "Total Number of Cycles"() -> (w542:dbl)
            n259 = call-poly <vilib>:"Read From Spreadsheet File.vi"("file path (dialog if empty)"=w545) -> ("first row"=w536:string[])  [unwired: 6 in, 4 out]
            n260 = call "Remove names.vi"("Array in"=w536) -> ("Array out"=w535:string[])  [unwired: 10 in]
            n261 = Number To Decimal String(number="Ageing Gas") -> (decimal integer string=w541:string)  [unwired: 1 in]
            n262 = Number To Decimal String(number=w542) -> (decimal integer string=w540:string)  [unwired: 1 in]
            n263 = Build Array (concatenate)(w541, w540, w535) -> (→"Ageing array":string[])
          }
        }
        "Cycle Compiled" <- w531
      }
      frame "convert to num" {
        n264 = local read "EditPos Subc"() -> (w551:T1)
        n265 = Unbundle By Name(w551) -> ("Row"=w552:i32, "Column"=w550:i32)
        n266 = Equal?(x=w550, y=7) -> (x = y?=w548:bool)
        n267 = case shown="False" w548 {
          tunnel: w552 -> [w557 _]
          tunnel: w550 -> [w555 _]
          frame False {
            n268 = local read "Subcycle Pattern"() -> (w554:string[][])
            n269 = call "Conv to num.vi"("Column"=w555, "Row"=w557, "Array"=w554) -> ("result string"=w556:string)  [unwired: 8 in]
            n270 = Replace Array Subset(array=w554, new element=w556, index (row)=w557, index (col)=w555) -> (w553:string[][])
            n271 = local write "Subcycle Pattern"(w553) -> ()
          }
          frame True {
          }
        }
      }
      frame "check scycle name" {
        n272 = local read "Subcycle name"() -> (w558:string)
        n273 = call <vilib>:"Search and Replace Pattern.vi"("string"=w558, "regular expression (\"\")"="[^0-9a-zA-Z ]" ("format string"), "replace string (\"\")"="", "replace all? (F)"=TRUE) -> ("result string"=w564:string)  [unwired: 1 in, 1 out]
        n274 = Not Equal?(x=w564, y=w558) -> (x != y?=w563:bool)
        n275 = case shown="False" w563 {
          tunnel: w564 -> [w565 w566]
          tunnel: [w565 w566] -> w559
          frame False {
          }
          frame True {
            n276 = One Button Dialog(message="Unsuitable character for the file name!") -> ()  [unwired: 1 in, 1 out]
          }
        }
        n277 = local write "Subcycle name"(w559) -> ()
      }
      frame "check cycle name" {
        n278 = local read "Cycle name"() -> (w568:string)
        n279 = call <vilib>:"Search and Replace Pattern.vi"("string"=w568, "regular expression (\"\")"="[^0-9a-zA-Z ]" ("format string"), "replace string (\"\")"="", "replace all? (F)"=TRUE) -> ("result string"=w574:string)  [unwired: 1 in, 1 out]
        n280 = Not Equal?(x=w574, y=w568) -> (x != y?=w573:bool)
        n281 = case shown="False" w573 {
          tunnel: w574 -> [w575 w576]
          tunnel: [w575 w576] -> w569
          frame False {
          }
          frame True {
            n282 = One Button Dialog(message="Unsuitable character for the file name!") -> ()  [unwired: 1 in, 1 out]
          }
        }
        n283 = local write "Cycle name"(w569) -> ()
      }
    }
    n284 = local read "stop"() -> (w33:bool)
  }
  n285 = while {
    tunnel: w27 -> [w582]
    shift-right: [w579] -> _
    shift-left: _ -> [w578]
    stop <- "stop" stop-if-true
    n286 = event shown="[12] \"Load cycle for test\": Value Change" {
      selector: _ -> [_ _ _ _ _ _ _ _ _ _ _ _ _ _ _]
      dyn-events: _ -> [_ _ _ _ _ _ _ _ _ _ _ _ _ _ _]
      timeout: 100 -> [_ _ _ _ _ _ _ _ _ _ _ _ _ _ _]
      tunnel: w582 -> [w585 w587 w591 w599 w606 w613 w623 w627 w637 w642 w645 w650 w672 w680 w681]
      tunnel: [w583 w586 w592 w598 w605 w612 w622 w625 w632 w639 w644 w648 w669 _ _] -> w579
      tunnel: w578 -> [w583 w586 w592 w598 w605 w611 w622 w625 w632 w639 w644 w648 w669 _ _]
      event Timeout {
        n287 = event-data() -> ()  [unwired: 1 in, 2 out]
        n288 = Enqueue Element(queue=w585, element=Control_3."main" ("Enum")) -> ()  [unwired: 2 in, 3 out]
      }
      event "Clear Pattern": Value Change {
        n289 = event-data() -> ()  [unwired: 1 in, 5 out]
        n290 = Enqueue Element(queue=w587, element=Control_3."clear table 1" ("Enum")) -> ()  [unwired: 2 in, 3 out]
      }
      event "Save Subcycle": Value Change {
        n291 = event-data() -> ()  [unwired: 1 in, 5 out]
        n292 = local read "Subcycle Pattern"() -> (w589:string[][])
        n293 = call "Time column check.vi"("Array"=w589) -> ("Mistake?"=w590:bool)  [unwired: 10 in]
        n294 = case shown="False" w590 {
          tunnel: w591 -> [w593 _]
          frame False {
            n295 = Enqueue Element(queue=w593, element=Control_3."save subc") -> (queue out=w595:refnum<queue>)  [unwired: 2 in, 2 out]
            n296 = Enqueue Element(queue=w595, element=Control_3."update list 1") -> ()  [unwired: 2 in, 3 out]
          }
          frame True {
            n297 = One Button Dialog(message="The time sequence is incorrect!\nReview and save again!") -> ()  [unwired: 1 in, 1 out]
          }
        }
      }
      event "Load Subcycle": Value Change {
        n298 = event-data() -> ()  [unwired: 1 in, 5 out]
        n299 = Enqueue Element(queue=w599, element=Control_3."load subc") -> ()  [unwired: 2 in, 3 out]
      }
      event "Delete Subcycle": Value Change {
        n300 = event-data() -> ()  [unwired: 1 in, 5 out]
        n301 = Enqueue Element(queue=w606, element=Control_3."delete subc") -> (queue out=w608:refnum<queue>)  [unwired: 2 in, 2 out]
        n302 = Enqueue Element(queue=w608, element=Control_3."update list 1") -> (queue out=w604:refnum<queue>)  [unwired: 2 in, 2 out]
        n303 = Enqueue Element(queue=w604, element=Control_3."update Cycle pattern ") -> (queue out=w601:refnum<queue>)  [unwired: 2 in, 2 out]
        n304 = Enqueue Element(queue=w601, element=Control_3."Total time calc") -> ()  [unwired: 2 in, 3 out]
      }
      event "Subcycle Pattern": Mouse Down; "Subcycle Pattern": Value Change {
        n305 = event-data() -> ()  [unwired: 1 in, 3 out]
        n306 = property on="Subcycle Pattern" class="Tbl (strict)"() -> ("EditPos"=w612:T1)  [unwired: 2 in, 2 out]
        n307 = Unbundle By Name(w612) -> ("Row"=w614:i32)  [unwired: 1 out]
        n308 = Less?(x=w614, y=30) -> (x < y?=w616:bool)
        n309 = case shown="True" w616 {
          tunnel: w613 -> [_ w621]
          frame False {
            n310 = One Button Dialog(message="This table is limited to 30 entries!") -> ()  [unwired: 1 in, 1 out]
          }
          frame True {
            n311 = Enqueue Element(queue=w621, element=Control_3."convert to num") -> (queue out=w620:refnum<queue>)  [unwired: 2 in, 2 out]
            n312 = Enqueue Element(queue=w620, element=Control_3."calc HC CO") -> ()  [unwired: 2 in, 3 out]
          }
        }
        "EditPos Subc" <- w611
        "Flag1" <- TRUE
      }
      event "Clear Pattern": Value Change {
        n313 = event-data() -> ()  [unwired: 1 in, 5 out]
        n314 = Enqueue Element(queue=w623, element=Control_3."clear table 2" ("Enum")) -> ()  [unwired: 2 in, 3 out]
      }
      event "Save Cycle": Value Change {
        n315 = event-data() -> ()  [unwired: 1 in, 5 out]
        n316 = Enqueue Element(queue=w627, element=Control_3."update Cycle pattern ") -> (queue out=w626:refnum<queue>)  [unwired: 2 in, 2 out]
        n317 = Enqueue Element(queue=w626, element=Control_3."save cycle") -> (queue out=w630:refnum<queue>)  [unwired: 2 in, 2 out]
        n318 = Enqueue Element(queue=w630, element=Control_3."update list 2") -> ()  [unwired: 2 in, 3 out]
      }
      event "Load Cycle": Value Change {
        n319 = event-data() -> ()  [unwired: 1 in, 5 out]
        n320 = Enqueue Element(queue=w637, element=Control_3."load cycle") -> (queue out=w635:refnum<queue>)  [unwired: 2 in, 2 out]
        n321 = Enqueue Element(queue=w635, element=Control_3."update Cycle pattern ") -> (queue out=w634:refnum<queue>)  [unwired: 2 in, 2 out]
        n322 = Enqueue Element(queue=w634, element=Control_3."Total time calc") -> ()  [unwired: 2 in, 3 out]
      }
      event "Delete Cycle": Value Change {
        n323 = event-data() -> ()  [unwired: 1 in, 5 out]
        n324 = Enqueue Element(queue=w642, element=Control_3."delete cycle") -> (queue out=w641:refnum<queue>)  [unwired: 2 in, 2 out]
        n325 = Enqueue Element(queue=w641, element=Control_3."update list 2") -> ()  [unwired: 2 in, 3 out]
      }
      event "Total Number of Cycles": Value Change {
        n326 = event-data() -> ()  [unwired: 1 in, 5 out]
        n327 = Enqueue Element(queue=w645, element=Control_3."Total time calc") -> ()  [unwired: 2 in, 3 out]
      }
      event "Cycle Pattern": Mouse Up; "Cycle Pattern": Value Change {
        n328 = event-data() -> ()  [unwired: 1 in, 3 out]
        n329 = property on="Cycle Pattern" class="Tbl (strict)"() -> ("EditPos"=w652:T1)  [unwired: 2 in, 2 out]
        n330 = Unbundle By Name(w652) -> ("Row"=w649:i32, "Column"=w654:i32)
        n331 = Less?(x=w649, y=30) -> (x < y?=w653:bool)
        n332 = case shown="True" w653 {
          tunnel: w654 -> [_ w656]
          tunnel: w650 -> [_ w659]
          frame False {
            n333 = One Button Dialog(message="This table is limited to 30 entries!") -> ()  [unwired: 1 in, 1 out]
          }
          frame True {
            n334 = Equal?(x=w656, y=1) -> (x = y?=w660:bool)
            n335 = case shown="True" w660 {
              tunnel: w659 -> [w663 w666]
              tunnel: [w662 w665] -> w658
              frame False {
                n336 = Enqueue Element(queue=w663, element=Control_3."update Cycle pattern ") -> (queue out=w662:refnum<queue>)  [unwired: 2 in, 2 out]
              }
              frame True {
                n337 = Enqueue Element(queue=w666, element=Control_3."load cycle name") -> (queue out=w665:refnum<queue>)  [unwired: 2 in, 2 out]
              }
            }
            n338 = Enqueue Element(queue=w658, element=Control_3."Total time calc") -> ()  [unwired: 2 in, 3 out]
          }
        }
        "Flag 2" <- TRUE
      }
      event "Load cycle for test": Value Change {
        n339 = event-data() -> ()  [unwired: 1 in, 5 out]
        n340 = local read "Flag 2"() -> (w668:bool)
        n341 = case shown="True" w668 {
          tunnel: w672 -> [w673 w677]
          tunnel: [w673 w674] -> w670
          frame False {
          }
          frame True {
            n342 = Enqueue Element(queue=w677, element=Control_3."save cycle") -> (queue out=w675:refnum<queue>)  [unwired: 2 in, 2 out]
            n343 = Enqueue Element(queue=w675, element=Control_3."update list 2") -> (queue out=w674:refnum<queue>)  [unwired: 2 in, 2 out]
          }
        }
        n344 = Enqueue Element(queue=w670, element=Control_3."load test array") -> ()  [unwired: 2 in, 3 out]
      }
      event "Subcycle name": Value Change {
        n345 = event-data() -> ()  [unwired: 1 in, 5 out]
        n346 = Enqueue Element(queue=w680, element=Control_3."check scycle name") -> ()  [unwired: 2 in, 3 out]
      }
      event "Cycle name": Value Change {
        n347 = event-data() -> ()  [unwired: 1 in, 5 out]
        n348 = Enqueue Element(queue=w681, element=Control_3."check cycle name") -> ()  [unwired: 2 in, 3 out]
      }
    }
  }
